vi "GFITS_VAR_ValHdrs.vi"(0 "action":T1(ring), 5 "header in":string[][](array[string]), 9 "data type":i32[](array[numeric]), 11 "error in (no error)":errorcluster) -> (6 "last headers":cluster{"ext":i32, "keywords":string[][]}[](array[cluster]), 15 "error out":errorcluster)   [LabVIEW 2016]
panel:
  out "headers":cluster{"ext":i32, "keywords":string[][]}[](array[cluster])
  in  "Cluster":cluster{"ext":i32, "keywords":string[][]}
  out "curr ext":string[][](array[string])
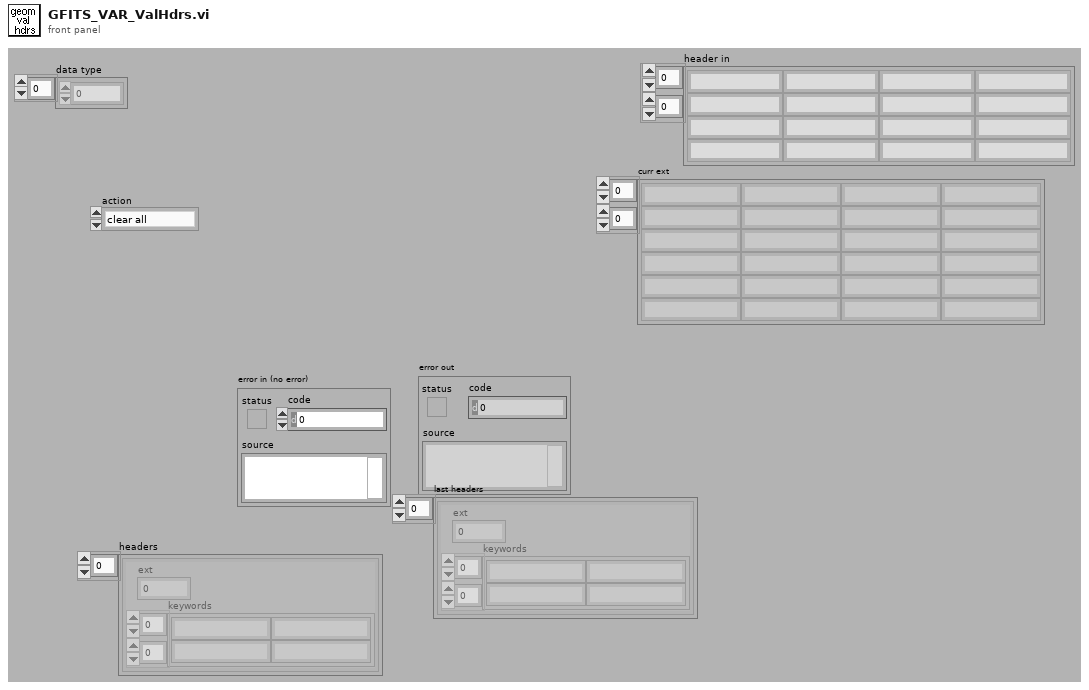
[diagram p1: front panel]
types:
  T1 = enum16{"clear all", "add extension", "add keyword", "get", "clear extension", "done"}
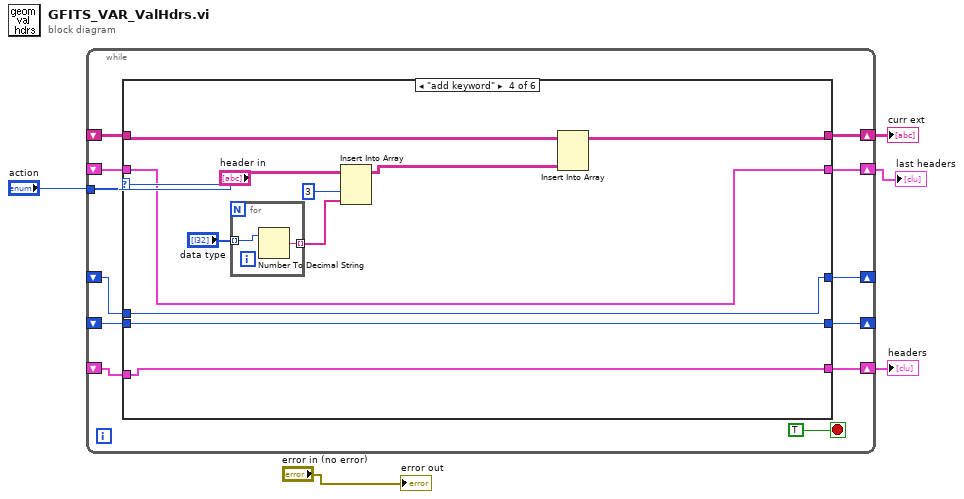
[diagram p0: block diagram]
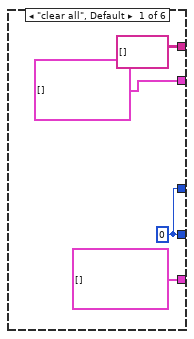
[diagram p2: hidden frame]
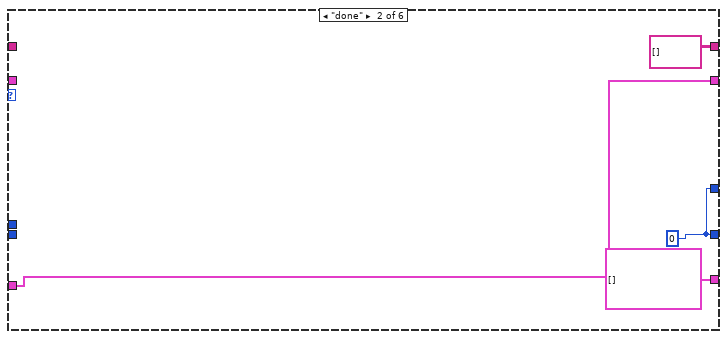
[diagram p3: hidden frame]
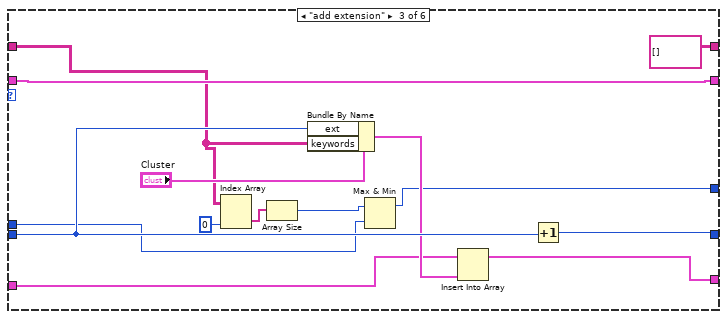
[diagram p4: hidden frame]
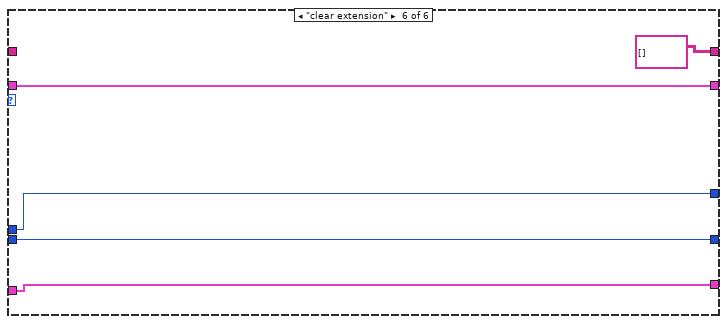
[diagram p6: hidden frame]
diagram:
  n1 = while {
    tunnel: "action" -> [w16]
    shift-right: [w15] -> w3
    shift-left: _ -> [w14]
    shift-right: [w13] -> w1
    shift-left: _ -> [w12]
    shift-right: [w8] -> w2
    shift-left: _ -> [w11]
    shift-right: [w10] -> _
    shift-left: _ -> [w9]
    shift-right: [w7] -> _
    shift-left: _ -> [w6]
    stop <- TRUE stop-if-true
    n2 = case shown="\"add keyword\"" w16 {
      tunnel: [string[][] [] ("GFITS_allkeys in") string[][] [] ("GFITS_allkeys in") string[][] [] ("GFITS_allkeys in") w45 w57 string[][] [] ("GFITS_allkeys in")] -> w15
      tunnel: w14 -> [_ _ w31 w46 w57 _]
      tunnel: [cluster{"ext":i32, "keywords":string[][]}[] [] w23 w38 w44 w53 w61] -> w13
      tunnel: w12 -> [_ _ w38 w44 w53 w61]
      tunnel: w11 -> [_ w23 w32 w41 w56 w59]
      tunnel: [w19 w24 w37 w42 w55 w60] -> w10
      tunnel: w9 -> [_ _ w36 w42 w55 w60]
      tunnel: [cluster{"ext":i32, "keywords":string[][]}[] [] cluster{"ext":i32, "keywords":string[][]}[] [] w33 w41 w56 w59] -> w8
      tunnel: [w19 w24 w26 w40 w54 w58] -> w7
      tunnel: w6 -> [_ _ w27 w40 w54 w58]
      frame "clear all", Default {
        w19 = 0
      }
      frame "done" {
        w24 = 0
      }
      frame "add extension" {
        n3 = Index Array(array=w31, index (col)=0 ("disabled index (col)")) -> (element=w29:string[])  [unwired: 1 in]
        n4 = Array Size(array=w29) -> (size(s)=w28:i32)
        n5 = Bundle By Name(cluster="Cluster", "ext"=w36, "keywords"=w31) -> (w34:cluster{"ext":i32, "keywords":string[][]})
        n6 = Max & Min(x=w28, y=w27) -> (max(x,y)=w26:i32)  [unwired: 1 out]
        n7 = Insert Into Array(array=w32, new element=w34) -> (w33:cluster{"ext":i32, "keywords":string[][]}[])  [unwired: 1 in]
        n8 = Increment(x=w36) -> (x+1=w37:i32)
      }
      frame "add keyword" {
        n9 = for {
          tunnel: "data type" -> [w52] mode=indexing
          tunnel: [w51] -> w49 mode=indexing
          n10 = Number To Decimal String(number=w52) -> (decimal integer string=w51:string)  [unwired: 1 out]
        }
        n11 = Insert Into Array(array="header in", index (col)=3 ("disabled index (col)"), new element=w49) -> (w43:string[][])  [unwired: 1 in]
        n12 = Insert Into Array(array=w46, new element=w43) -> (w45:string[][])  [unwired: 2 in]
      }
      frame "get" {
      }
      frame "clear extension" {
      }
    }
  }
  "curr ext" <- w3
  "headers" <- w2
  "last headers" <- w1
  "error out" <- "error in (no error)"
